vi "Configure Serial Bus (NRZ - Basic).vi"(0 "VISA resource name":refnum<visa-resource-name>, 1 "Idle State (0: Low)":i32(ring) items=["Low", "High"], 2 "Start Bit (1)":i32=1, 5 "Serial Bus Name (1: Serial Bus 1)":i32(ring)=1 items=["Serial Bus 1"=1, "Serial Bus 2"=2], 7 "Source Channel (0: Channel 1)":i32(ring) items=["Channel 1", "Channel 2", "Channel 3", "Channel 4", "D0", "D1", "D2", "D3", "D4", "D5", "D6", "D7", "D8", "D9", "D10", "D11", "D12", "D13", "D14", "D15"], 9 "Logic 1 (0: High)":i32(ring) items=["High", "Low"], 11 "error in (no error)":errorcluster, 12 "Baud Rate (125000 bps)":i32=125000, 13 "Idle Time (10)":dbl=10.0) -> (4 "VISA resource name out":refnum<visa-resource-name>, 15 "error out":errorcluster)   [LabVIEW 2015, in "Agilent 2000 3000 X-Series.lvlib"]
doc: "Configures the basic setting of NRZ bus.\n\n<b>Note:</b>\nThis VI is only applicable for 3000T, 4000, 6000 X-Series."
uses:
  Agilent 2000 3000 X-Series.lvlib
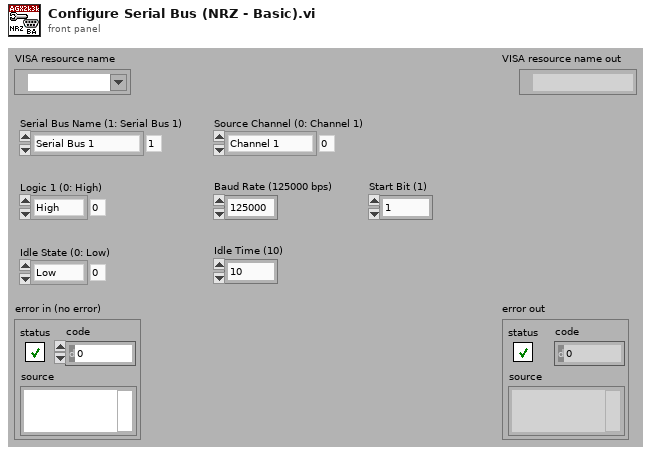
[diagram p1: front panel]
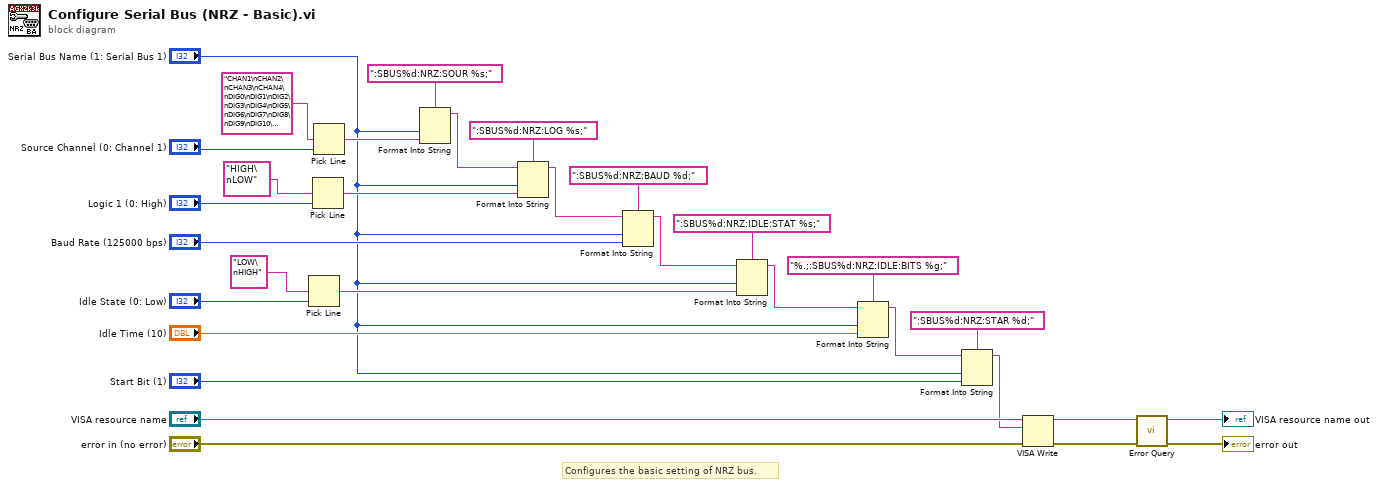
[diagram p0: block diagram]
diagram:
  # "Configures the basic setting of NRZ bus."
  n1 = Pick Line(multi-line string="LOW\nHIGH", line index="Idle State (0: Low)") -> (output string=w24:string)  [unwired: 1 in]
  n2 = Pick Line(multi-line string="HIGH\nLOW", line index="Logic 1 (0: High)") -> (output string=w20:string)  [unwired: 1 in]
  n3 = Pick Line(multi-line string="CHAN1\nCHAN2\nCHAN3\nCHAN4\nDIG0\nDIG1\nDIG2\nDIG3\nDIG4\nDIG5\nDIG6\nDIG7\nDIG8\nDIG9\nDIG10\nDIG11\nDIG12\nDIG13\nDIG14\nDIG15", line index="Source Channel (0: Channel 1)") -> (output string=w16:string)  [unwired: 1 in]
  n4 = Format Into String(format string=":SBUS%d:NRZ:SOUR %s;", "Serial Bus Name (1: Serial Bus 1)", w16) -> (resulting string=w11:string)  [unwired: 2 in, 1 out]
  n5 = Format Into String(format string=":SBUS%d:NRZ:LOG %s;", initial string=w11, "Serial Bus Name (1: Serial Bus 1)", w20) -> (resulting string=w10:string)  [unwired: 1 in, 1 out]
  n6 = Format Into String(format string=":SBUS%d:NRZ:BAUD %d;", initial string=w10, "Serial Bus Name (1: Serial Bus 1)", "Baud Rate (125000 bps)") -> (resulting string=w9:string)  [unwired: 1 in, 1 out]
  n7 = Format Into String(format string=":SBUS%d:NRZ:IDLE:STAT %s;", initial string=w9, "Serial Bus Name (1: Serial Bus 1)", w24) -> (resulting string=w8:string)  [unwired: 1 in, 1 out]
  n8 = Format Into String(format string="%.;:SBUS%d:NRZ:IDLE:BITS %g;", initial string=w8, "Serial Bus Name (1: Serial Bus 1)", "Idle Time (10)") -> (resulting string=w6:string)  [unwired: 1 in, 1 out]
  n9 = Format Into String(format string=":SBUS%d:NRZ:STAR %d;", initial string=w6, "Serial Bus Name (1: Serial Bus 1)", "Start Bit (1)") -> (resulting string=w1:string)  [unwired: 1 in, 1 out]
  n10 = VISA Write(VISA resource name="VISA resource name", write buffer=w1, error in (no error)="error in (no error)") -> (VISA resource name out=w5:refnum<visa-resource-name>, error out=w4:errorcluster)  [unwired: 1 out]
  n11 = call "Error Query.vi"("error in (no error)"=w4, "VISA resource name"=w5) -> ("error out"=→"error out":errorcluster, "VISA resource name out"=→"VISA resource name out":refnum<visa-resource-name>)  [unwired: 6 in, 2 out]
